vi "NTU Read Pin Map.vi"(8 "error in (no error)":errorcluster, 11 "NI-DAQ in":refnum<class "Copy of NI-DAQ.lvclass">) -> (0 "error out":errorcluster, 2 "Pin Map":T1={"Region Valves"=[49, 52, 0, 0], "Extra Valves"=[[0.0, 48.0, 0.0, 0.0, 0.0]], "Tool Primary Valve"=51, "Tool Secondary Valve"=50, "Region Sensors"=[37, 41, 37], "Extra Sensors"=[[36.0, 37.0, 0.0, 0.0]], "Tool Primary Sensor"=39.0, "Tool Secondary Sensor"=38.0, "Compression Sensor"=31.0, "5V"=50, "NTU_Glue"=0.0}, 3 "NI-DAQ out":refnum<class "Copy of NI-DAQ.lvclass">)   [LabVIEW 2016]
uses:
  HGCal Software/Gantry Software/V5/Classes/Controller/I-O/Pin Map.ctl
  HGCal Software/Gantry Software/V5/Classes/Controller/I-O/I-O.lvclass
  Copy of NI-DAQ.lvclass
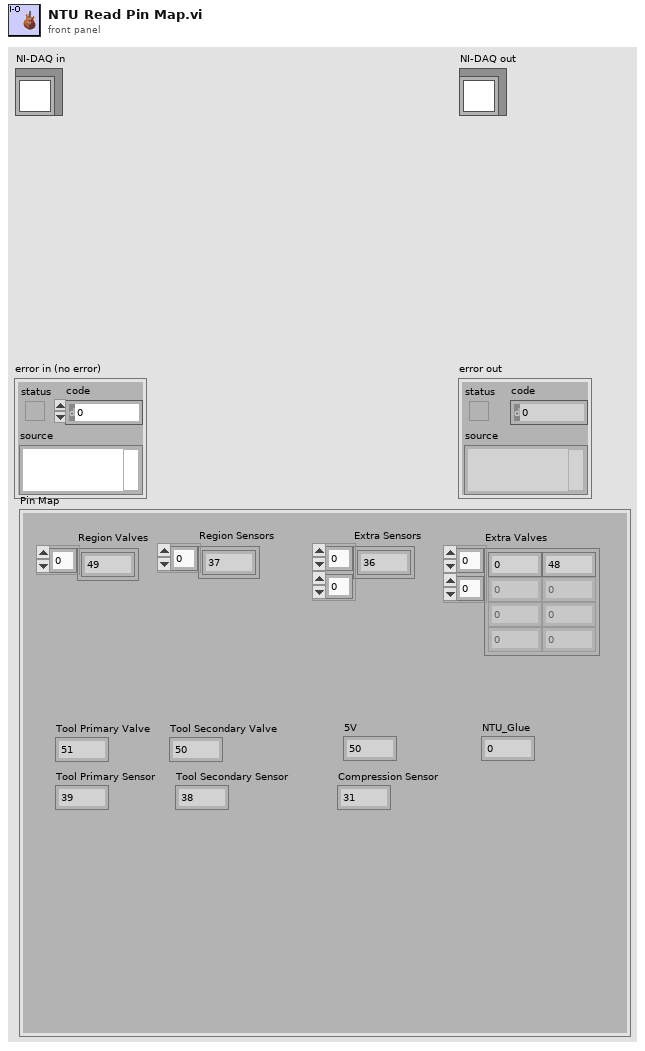
[diagram p1: front panel]
types:
  T1 = typedef "I-O.lvclass/Pin Map.ctl" = cluster{"Region Valves":i32[], "Extra Valves":dbl[][], "Tool Primary Valve":i32, "Tool Secondary Valve":i32, "Region Sensors":i32[], "Extra Sensors":dbl[][], "Tool Primary Sensor":dbl, "Tool Secondary Sensor":dbl, "Compression Sensor":dbl, "5V":i32, "NTU_Glue":dbl}
  T2 = typedef "Copy of I-O.lvclass/Pin Map.ctl" = cluster{"Region Valves":i32[], "Extra Valves":dbl[][], "Tool Primary Valve":i32, "Tool Secondary Valve":i32, "Region Sensors":i32[], "Extra Sensors":dbl[][], "Tool Primary Sensor":dbl, "Tool Secondary Sensor":dbl, "Compression Sensor":dbl, "5V":i32, "NTU_Glue":dbl}
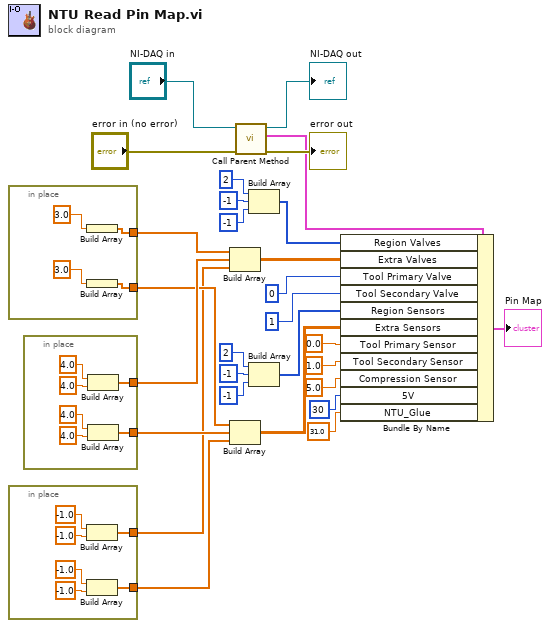
[diagram p0: block diagram]
diagram:
  n1 = in-place {
    in-place-border: [w31] -> w18
    in-place-border: [w30] -> w15
    n2 = Build Array(3.0 ("element")) -> (w31:dbl[])
    n3 = Build Array(3.0 ("element")) -> (w30:dbl[])
  }
  n4 = in-place {
    in-place-border: [w37] -> w4
    in-place-border: [w36] -> w3
    n5 = Build Array(-1.0 ("element"), -1.0 ("element")) -> (w37:dbl[])
    n6 = Build Array(-1.0 ("element"), -1.0 ("element")) -> (w36:dbl[])
  }
  n7 = in-place {
    in-place-border: [w43] -> w17
    in-place-border: [w42] -> w14
    n8 = Build Array(4.0 ("element"), 4.0 ("element")) -> (w43:dbl[])
    n9 = Build Array(4.0 ("element"), 4.0 ("element")) -> (w42:dbl[])
  }
  n10 = Build Array(w18, w17, w4) -> (w16:dbl[][])
  n11 = Build Array(w15, w14, w3) -> (w13:dbl[][])
  n12 = call-parent "Call Parent Method"("error in (no error)"="error in (no error)", "I-O in"="NI-DAQ in") -> ("error out"=→"error out":errorcluster, "Pin Map"=w25:T2, "I-O out"=→"NI-DAQ out":refnum<class "Copy of NI-DAQ.lvclass">)  [unwired: 7 in]
  n13 = Build Array(i16 2 ("element"), i16 -1 ("element"), i16 -1 ("element")) -> (w7:i16[])
  n14 = Build Array(i16 2 ("element"), i16 -1 ("element"), i16 -1 ("element")) -> (w12:i16[])
  n15 = Bundle By Name(cluster=w25, "Region Valves"=w7, "Extra Valves"=w16, "Tool Primary Valve"=0, "Tool Secondary Valve"=1, "Region Sensors"=w12, "Extra Sensors"=w13, "Tool Primary Sensor"=0.0, "Tool Secondary Sensor"=1.0, "Compression Sensor"=5.0, "5V"=30, "NTU_Glue"=31.0) -> (→"Pin Map":T2)
